vi "DynamicMotionMagicExpoTorqueCurrentFOC SetControl.vi"(0 "DeviceReference":T1, 1 "Position":dbl, 2 "kV":dbl, 3 "kA":dbl, 4 "Velocity":dbl, 5 "FeedForward":dbl, 6 "Slot":i32, 7 "error in":errorcluster, 8 "OverrideCoastDurNeutral":bool, 9 "LimitForwardMotion":bool, 10 "LimitReverseMotion":bool, 11 "IgnoreHardwareLimits":bool, 12 "IgnoreSoftwareLimits":bool, 13 "UseTimesync":bool, 18 "Update Frequency (Hz)":dbl=100.0) -> (20 "DeviceReference Out":T1, 27 "error out":errorcluster)   [LabVIEW 2025]
doc: "Requests Motion Magic® Expo to target a final position using an exponential motion profile. This dynamic request allows runtime changes to the profile kV, kA, and (optional) Cruise Velocity. Users can optionally provide a torque current feedforward.\nMotion Magic® Expo produces a motion profile in real-time while attempting to honor the specified Cruise Velocity (optional) and the mechanism kV and kA. Note that unlike the slot gains, the Expo_kV and Expo_kA parameters are always in output units of Volts.\nSetting the Cruise Velocity to 0 will allow the profile to run to the max possible velocity based on Expo_kV. This control mode does not use the Acceleration or Jerk configs.\nTarget position can be changed on-the-fly and Motion Magic® will do its best to adjust the profile. This control mode is based on torque current, so relevant closed-loop gains will use Amperes for the numerator."
uses:
  <vilib>/Rock Robotics/WPI/ThirdParty/Phoenix6/DeviceReference.ctl
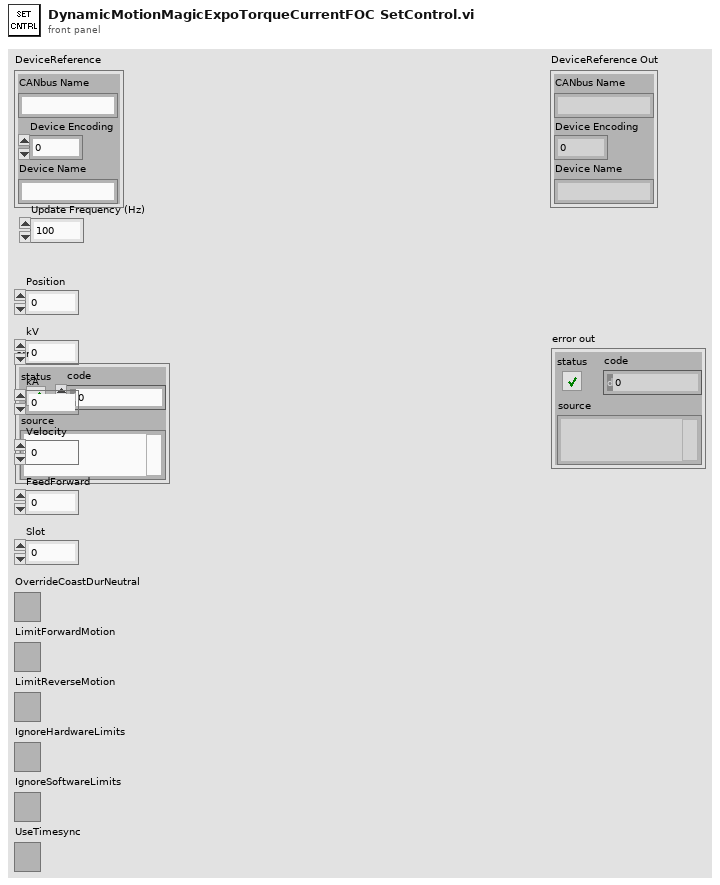
[diagram p1: front panel]
types:
  T1 = typedef "DeviceReference.ctl" = cluster{"CANbus Name":string, "Device Encoding":u32, "Device Name":string}
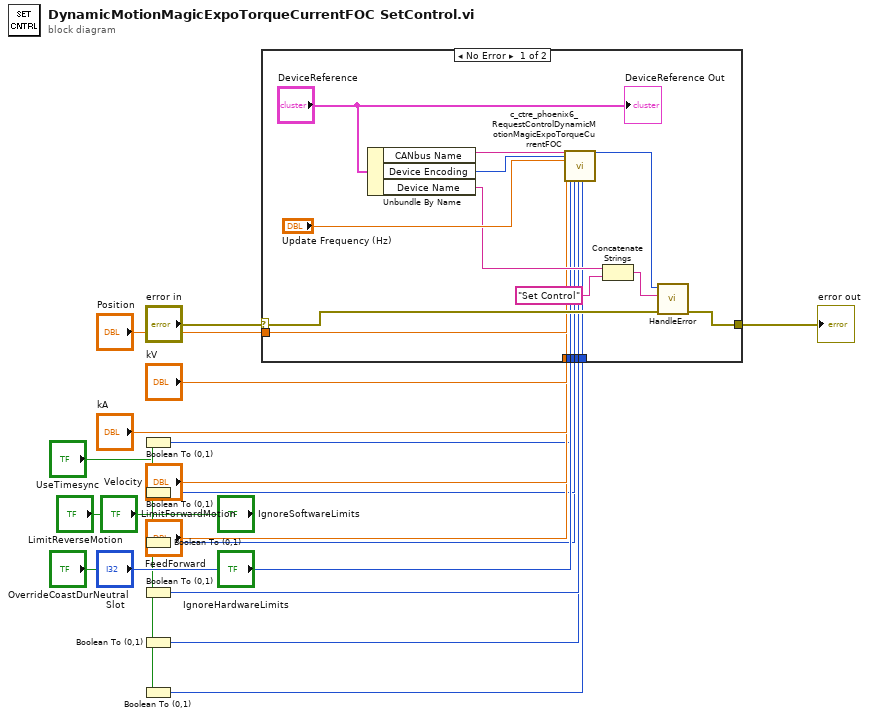
[diagram p0: block diagram]
diagram:
  n1 = Boolean To (0,1)(Boolean="OverrideCoastDurNeutral") -> (0, 1=w11:i16)
  n2 = Boolean To (0,1)(Boolean="LimitForwardMotion") -> (0, 1=w9:i16)
  n3 = Boolean To (0,1)(Boolean="LimitReverseMotion") -> (0, 1=w7:i16)
  n4 = Boolean To (0,1)(Boolean="IgnoreHardwareLimits") -> (0, 1=w5:i16)
  n5 = Boolean To (0,1)(Boolean="IgnoreSoftwareLimits") -> (0, 1=w3:i16)
  n6 = Boolean To (0,1)(Boolean="UseTimesync") -> (0, 1=w1:i16)
  n7 = case shown="No Error" "error in" {
    selector: "error in" -> [w37 w43]
    tunnel: [w36 w43] -> w19
    tunnel: "Position" -> [w32 _]
    tunnel: "kV" -> [w31 _]
    tunnel: "kA" -> [w30 _]
    tunnel: "Velocity" -> [w29 _]
    tunnel: "FeedForward" -> [w28 _]
    tunnel: "Slot" -> [w27 _]
    tunnel: w11 -> [w26 _]
    tunnel: w9 -> [w25 _]
    tunnel: w7 -> [w24 _]
    tunnel: w5 -> [w23 _]
    tunnel: w3 -> [w22 _]
    tunnel: w1 -> [w21 _]
    frame No Error {
      n8 = Unbundle By Name("DeviceReference") -> ("CANbus Name"=w41:string, "Device Encoding"=w40:u32, "Device Name"=w35:string)
      n9 = call <vilib>:"c_ctre_phoenix6_RequestControlDynamicMotionMagicExpoTorqueCurrentFOC.vi"("String 2"=w41, "Numeric 2"=w40, "Numeric 3"="Update Frequency (Hz)", "Numeric 4"=w32, "Numeric 5"=w31, "Numeric 6"=w30, "Numeric 7"=w29, "Numeric 8"=w28, "Numeric 9"=w27, "Numeric 10"=w26, "Numeric 11"=w25, "Numeric 12"=w24, "Numeric 13"=w23, "Numeric 14"=w22, "Numeric 15"=w21) -> ("Numeric"=w38:i32)  [unwired: 11 in, 1 out]
      n10 = Concatenate Strings(w35, "Set Control" ("origin")) -> (w33:string)
      n11 = call <vilib>:"HandleError.vi"("error in"=w37, "origin"=w33, "Status"=w38) -> ("error out"=w36:errorcluster)  [unwired: 8 in]
      "DeviceReference Out" <- "DeviceReference"
    }
    frame Error {
    }
  }
  "error out" <- w19
